vi "ShowOnlyMatches.vi"(8 "error in (no error)":errorcluster, 10 "IP Stats In":T1[](array[typedef])) -> (0 "error out":errorcluster, 2 "IP Stats Out":T1[](array[typedef]))   [LabVIEW 2020, in "Controller.lvlib"]
uses:
  Controller.lvlib
  Public Controls/IP Stats.ctl
  UI/UI.lvlib
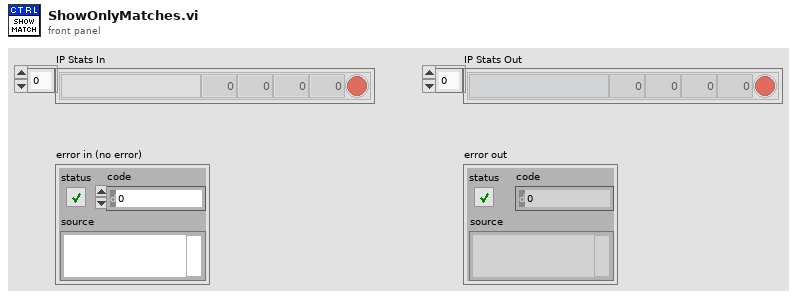
[diagram p1: front panel]
types:
  T1 = typedef "UI.lvlib/IP Stats.ctl" = cluster{"Address":string, "Average Response Time":i32, "Loss %":i32, "Min Response Time":i32, "Max Response Time":i32, "Boolean":bool}
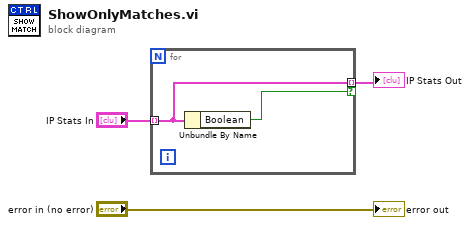
[diagram p0: block diagram]
diagram:
  n1 = for {
    tunnel: "IP Stats In" -> [w5] mode=indexing
    tunnel: [w5] -> w2 mode=indexing if=w4
    n2 = Unbundle By Name(w5) -> ("Boolean"=w4:bool)
  }
  "IP Stats Out" <- w2
  "error out" <- "error in (no error)"
